vi "UDT_application_Get Data Out.vi"() -> (3 "Unit Test Framework Results":T1)   [LabVIEW 2017]
doc: "Use this template to create a user-defined test VI. Define your test requirements and wire the results to the <b>Result (Test)</b> control. Do not modify the <b>Unit Test Framework Results</b> indicator."
uses:
  <vilib>/utf/common/utf_test_result_troll.ctl
  <vilib>/utf/common/utf_test_result.ctl
  <vilib>/utf/common/utf_test_result_failure.ctl
  <vilib>/utf/common/utf_test_comparison_operators.ctl
  <vilib>/utf/common/utf_vi_tag.ctl
  RT/TypeDefs/dataOut.ctl
  RT/TypeDefs/allData.ctl
  RT/TypeDefs/dataIn.ctl
  RT/SubVIs/FGVs/TypeDefs/DataFGVControl.ctl
  <vilib>/Control Software Solutions Ltd/UTF Helper/SubVIs/UTF Boolean Equals.vi
  <vilib>/Control Software Solutions Ltd/UTF Helper/SubVIs/UTF Double Equals.vi
  <vilib>/Control Software Solutions Ltd/UTF Helper/SubVIs/UTF I32 Equals.vi
  <vilib>/Control Software Solutions Ltd/UTF Helper/Unit Test Helper.lvlib
  <vilib>/utf/NI_UnitTestFramework.lvlib
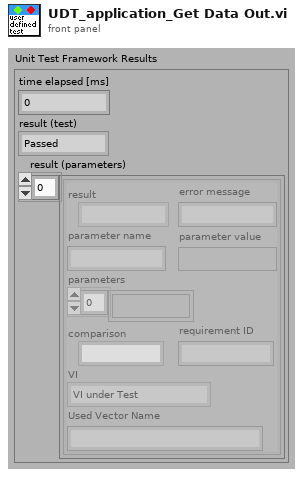
[diagram p1: front panel]
types:
  T1 = typedef "NI_UnitTestFramework.lvlib/utf_test_result_troll.ctl" = cluster{"time elapsed [ms]":u32, "result (test)":T2, "result (parameters)":T3[]}
  T2 = typedef "NI_UnitTestFramework.lvlib/utf_test_result.ctl" = enum16{"Passed", "Failed", "Error", "Skipped", "Not Processed"}
  T3 = typedef "NI_UnitTestFramework.lvlib/utf_test_result_failure.ctl" = cluster{"result":T2, "error message":string, "parameter name":string, "parameter value":variant, "parameters":variant[], "comparison":T4, "requirement ID":string, "VI":T5, "Used Vector Name":string}
  T4 = typedef "NI_UnitTestFramework.lvlib/utf_test_comparison_operators.ctl" = enum16{"=", "!=", ">", ">=", "<", "<=", "range", "symmetric tolerance", "asymmetric tolerance", "string contains", "string not contain", "array size", "string length", "array range", "by element", "array range (limit array)", "user-defined", "array contains", "array not contain", "vector length", "= (elm)", "!= (elm)", "= (case insensitive)", "!= (case insensitive)"}
  T5 = typedef "NI_UnitTestFramework.lvlib/utf_vi_tag.ctl" = enum16{"Setup VI", "VI under Test", "Teardown VI"}
  T6 = typedef "DataFGVControl.ctl" = enum16{"Set Data", "Get Data"}
  T7 = typedef "allData.ctl" = cluster{"DataOut":T8, "DataIn":T9}
  T8 = typedef "dataOut.ctl" = cluster{"X0pos":dbl, "Y0pos":dbl, "Z0pos":dbl, "Fx":dbl, "Fy":dbl, "Fz":dbl, "Encoder1":i32, "Encoder2":i32, "Pot1":dbl, "Pot2":dbl, "Theta0":dbl, "Theta1":dbl, "X1pos":dbl, "Y1pos":dbl, "Z1pos":dbl, "X2pos":dbl, "Y2pos":dbl, "Z2pos":dbl, "ErrorOccurred":bool}
  T9 = typedef "dataIn.ctl" = cluster{"Xtarget":dbl, "Ytarget":dbl, "Ztarget":dbl, "X_Attractor 1":dbl, "Y_Attractor 1":dbl, "Z_Attractor 1":dbl, "X_Attractor 2":dbl, "Y_Attractor 2":dbl, "Z_Attractor 2":dbl, "Traj Flag":bool, "DeadZone":dbl, "Assistance":bool, "Shutdown?":bool, "AssistanceLevel":dbl}
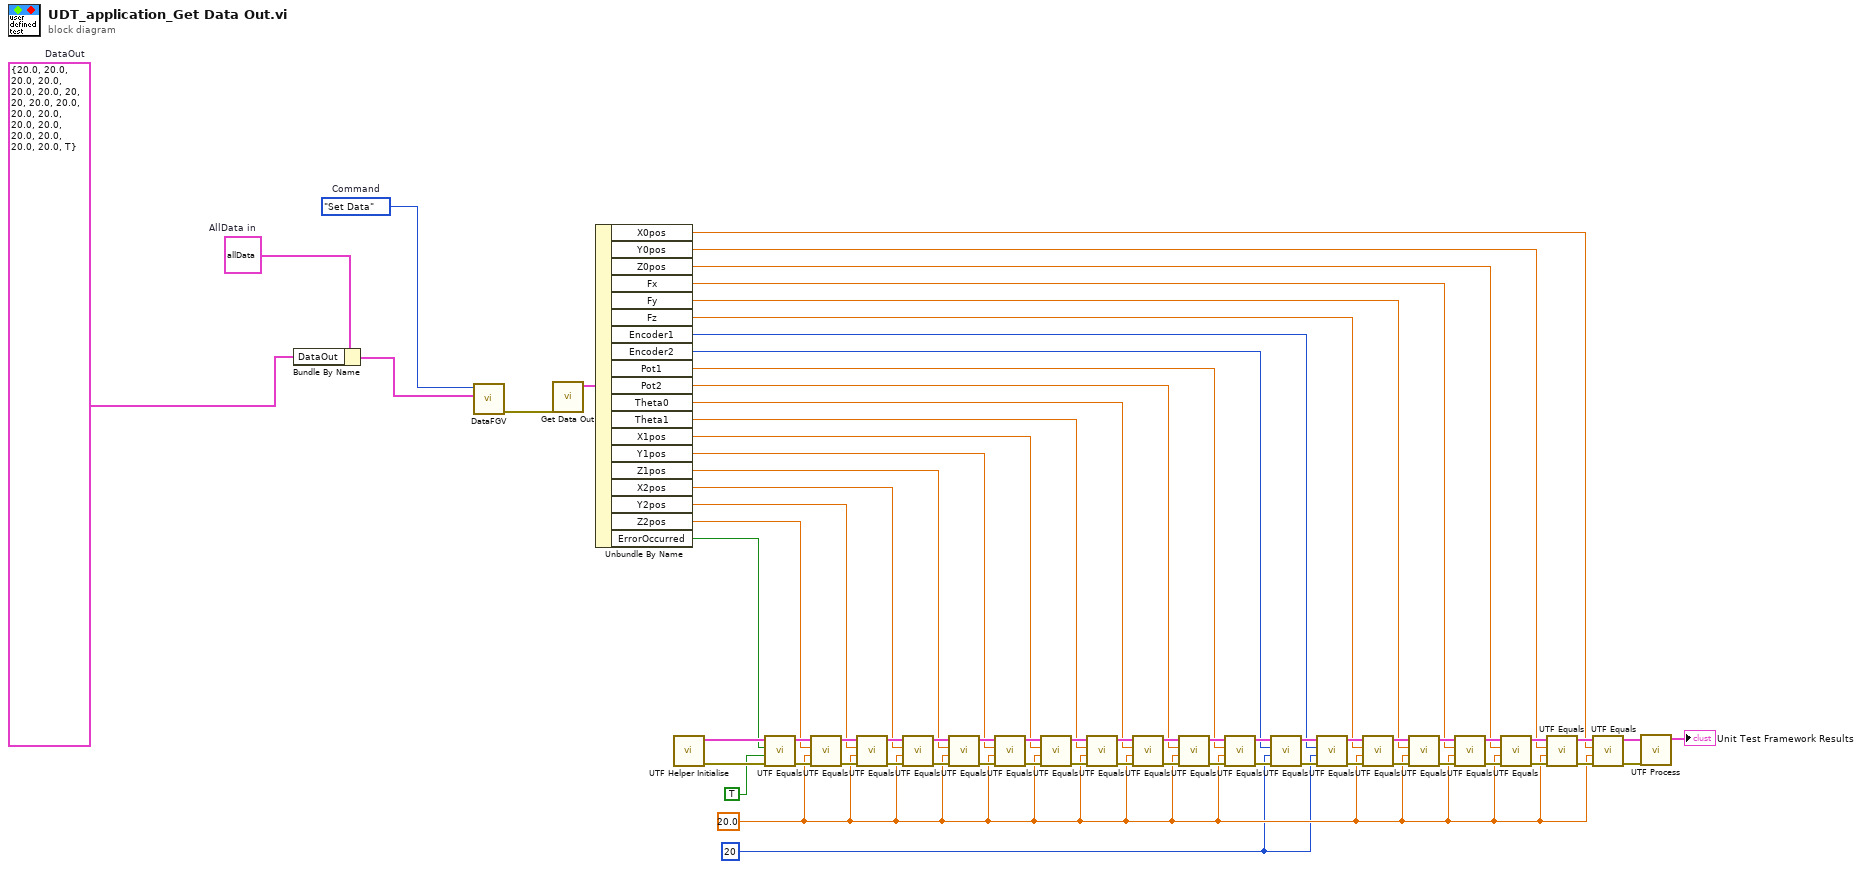
[diagram p0: block diagram]
diagram:
  w1 = DataFGVControl."Set Data"  # Command
  w4 = T7 {"DataOut"={"X0pos"=0.0, "Y0pos"=0.0, "Z0pos"=0.0, "Fx"=0.0, "Fy"=0.0, "Fz"=0.0, "Encoder1"=0, "Encoder2"=0, "Pot1"=0.0, "Pot2"=0.0, "Theta0"=0.0, "Theta1"=0.0, "X1pos"=0.0, "Y1pos"=0.0, "Z1pos"=0.0, "X2pos"=0.0, "Y2pos"=0.0, "Z2pos"=0.0, "ErrorOccurred"=FALSE}, "DataIn"={"Xtarget"=0.0, "Ytarget"=0.0, "Ztarget"=0.0, "X_Attractor 1"=0.0, "Y_Attractor 1"=0.0, "Z_Attractor 1"=0.0, "X_Attractor 2"=0.0, "Y_Attractor 2"=0.0, "Z_Attractor 2"=0.0, "Traj Flag"=FALSE, "DeadZone"=0.0, "Assistance"=FALSE, "Shutdown?"=FALSE, "AssistanceLevel"=0.0}}  # AllData in
  w3 = T8 {"X0pos"=20.0, "Y0pos"=20.0, "Z0pos"=20.0, "Fx"=20.0, "Fy"=20.0, "Fz"=20.0, "Encoder1"=20, "Encoder2"=20, "Pot1"=20.0, "Pot2"=20.0, "Theta0"=20.0, "Theta1"=20.0, "X1pos"=20.0, "Y1pos"=20.0, "Z1pos"=20.0, "X2pos"=20.0, "Y2pos"=20.0, "Z2pos"=20.0, "ErrorOccurred"=TRUE}  # DataOut
  w27 = 20 ("Encoder2")
  w28 = 20.0 ("Z2pos")
  n1 = Bundle By Name(cluster=w4, "DataOut"=w3) -> (w2:T7)
  n2 = call "DataFGV.vi"("AllData in"=w2, "Command"=w1) -> ("error out"=w5:errorcluster)  [unwired: 8 in, 1 out]
  n3 = call "Get Data Out.vi"("error in (no error)"=w5) -> ("DataOut"=w25:T8)  [unwired: 9 in, 1 out]
  n4 = Unbundle By Name(w25) -> ("X0pos"=w6:dbl, "Y0pos"=w7:dbl, "Z0pos"=w8:dbl, "Fx"=w9:dbl, "Fy"=w10:dbl, "Fz"=w11:dbl, "Encoder1"=w12:i32, "Encoder2"=w13:i32, "Pot1"=w14:dbl, "Pot2"=w15:dbl, "Theta0"=w16:dbl, "Theta1"=w17:dbl, "X1pos"=w18:dbl, "Y1pos"=w19:dbl, "Z1pos"=w20:dbl, "X2pos"=w21:dbl, "Y2pos"=w22:dbl, "Z2pos"=w23:dbl, "ErrorOccurred"=w24:bool)
  n5 = call <vilib>:"UTF Helper Initialise.vi"() -> ("error out"=w68:errorcluster, "results array"=w69:T3[])  [unwired: 10 in]
  n6 = call-poly <vilib>:"UTF Equals.vi"("error in (no error)"=w68, "Test Value"=TRUE, "Input"=w24, "Input Results"=w69) -> ("error out"=w67:errorcluster, "Output Results"=w66:T3[])  [unwired: 6 in]
  n7 = call-poly <vilib>:"UTF Equals.vi"("error in (no error)"=w67, "Test Value"=w28, "Input"=w23, "Input Results"=w66) -> ("error out"=w65:errorcluster, "Output Results"=w64:T3[])  [unwired: 6 in]
  n8 = call-poly <vilib>:"UTF Equals.vi"("error in (no error)"=w65, "Test Value"=w28, "Input"=w22, "Input Results"=w64) -> ("error out"=w63:errorcluster, "Output Results"=w62:T3[])  [unwired: 6 in]
  n9 = call-poly <vilib>:"UTF Equals.vi"("error in (no error)"=w63, "Test Value"=w28, "Input"=w21, "Input Results"=w62) -> ("error out"=w61:errorcluster, "Output Results"=w60:T3[])  [unwired: 6 in]
  n10 = call-poly <vilib>:"UTF Equals.vi"("error in (no error)"=w61, "Test Value"=w28, "Input"=w20, "Input Results"=w60) -> ("error out"=w59:errorcluster, "Output Results"=w58:T3[])  [unwired: 6 in]
  n11 = call-poly <vilib>:"UTF Equals.vi"("error in (no error)"=w59, "Test Value"=w28, "Input"=w19, "Input Results"=w58) -> ("error out"=w34:errorcluster, "Output Results"=w46:T3[])  [unwired: 6 in]
  n12 = call-poly <vilib>:"UTF Equals.vi"("error in (no error)"=w34, "Test Value"=w28, "Input"=w18, "Input Results"=w46) -> ("error out"=w53:errorcluster, "Output Results"=w52:T3[])  [unwired: 6 in]
  n13 = call-poly <vilib>:"UTF Equals.vi"("error in (no error)"=w53, "Test Value"=w28, "Input"=w17, "Input Results"=w52) -> ("error out"=w54:errorcluster, "Output Results"=w47:T3[])  [unwired: 6 in]
  n14 = call-poly <vilib>:"UTF Equals.vi"("error in (no error)"=w54, "Test Value"=w28, "Input"=w16, "Input Results"=w47) -> ("error out"=w55:errorcluster, "Output Results"=w45:T3[])  [unwired: 6 in]
  n15 = call-poly <vilib>:"UTF Equals.vi"("error in (no error)"=w55, "Test Value"=w28, "Input"=w15, "Input Results"=w45) -> ("error out"=w56:errorcluster, "Output Results"=w44:T3[])  [unwired: 6 in]
  n16 = call-poly <vilib>:"UTF Equals.vi"("error in (no error)"=w56, "Test Value"=w28, "Input"=w14, "Input Results"=w44) -> ("error out"=w57:errorcluster, "Output Results"=w43:T3[])  [unwired: 6 in]
  n17 = call-poly <vilib>:"UTF Equals.vi"("error in (no error)"=w57, "Test Value"=w27, "Input"=w13, "Input Results"=w43) -> ("error out"=w35:errorcluster, "Output Results"=w36:T3[])  [unwired: 6 in]
  n18 = call-poly <vilib>:"UTF Equals.vi"("error in (no error)"=w35, "Test Value"=w27, "Input"=w12, "Input Results"=w36) -> ("error out"=w51:errorcluster, "Output Results"=w42:T3[])  [unwired: 6 in]
  n19 = call-poly <vilib>:"UTF Equals.vi"("error in (no error)"=w51, "Test Value"=w28, "Input"=w11, "Input Results"=w42) -> ("error out"=w50:errorcluster, "Output Results"=w41:T3[])  [unwired: 6 in]
  n20 = call-poly <vilib>:"UTF Equals.vi"("error in (no error)"=w50, "Test Value"=w28, "Input"=w10, "Input Results"=w41) -> ("error out"=w49:errorcluster, "Output Results"=w40:T3[])  [unwired: 6 in]
  n21 = call-poly <vilib>:"UTF Equals.vi"("error in (no error)"=w49, "Test Value"=w28, "Input"=w9, "Input Results"=w40) -> ("error out"=w48:errorcluster, "Output Results"=w39:T3[])  [unwired: 6 in]
  n22 = call-poly <vilib>:"UTF Equals.vi"("error in (no error)"=w48, "Test Value"=w28, "Input"=w8, "Input Results"=w39) -> ("error out"=w37:errorcluster, "Output Results"=w38:T3[])  [unwired: 6 in]
  n23 = call-poly <vilib>:"UTF Equals.vi"("error in (no error)"=w37, "Test Value"=w28, "Input"=w7, "Input Results"=w38) -> ("error out"=w33:errorcluster, "Output Results"=w32:T3[])  [unwired: 6 in]
  n24 = call-poly <vilib>:"UTF Equals.vi"("error in (no error)"=w33, "Test Value"=w28, "Input"=w6, "Input Results"=w32) -> ("error out"=w31:errorcluster, "Output Results"=w30:T3[])  [unwired: 6 in]
  n25 = call <vilib>:"UTF Process.vi"("error in (no error)"=w31, "results array"=w30) -> ("Unit Test Framework Results"=→"Unit Test Framework Results":T1)  [unwired: 9 in]
